vi "launch connection handler.vi"(7 "TCP Network Connection Refnum":refnum<k5>, 8 "error in":errorcluster, 9 "to application":refnum<queue>, 10 "to listener":refnum<queue>, 11 "VI ref":variant) -> (0 "error IO":errorcluster, 3 "to handler":refnum<queue>)   [LabVIEW 2015]
uses:
  message/message.ctl
  message/message type.lvlib
  TCP connection/TCP connection.lvclass
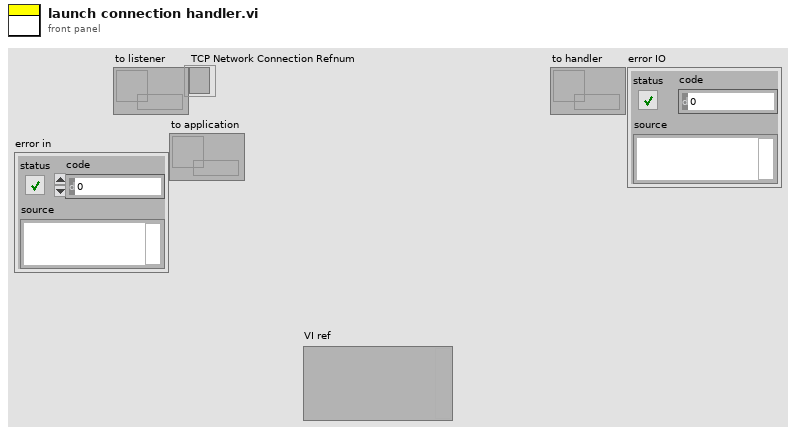
[diagram p1: front panel]
types:
  T1 = typedef "message type.lvlib/message.ctl" = cluster{"ID":string, "data":variant}
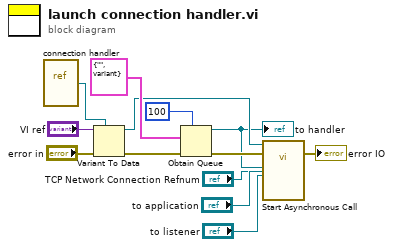
[diagram p0: block diagram]
diagram:
  n1 = vi-ref "connection handler.vi"() -> (w8:refnum<vi>)
  n2 = Variant To Data(error in="error in", type=w8, Variant="VI ref") -> (data=w6:refnum<vi>, error out=w9:errorcluster)
  n3 = Obtain Queue(max queue size (-1, unlimited)=100, element data type=T1 {"ID"="", "data"=variant} ("message"), error in (no error)=w9) -> (queue out=w5:refnum<queue>, error out=w11:errorcluster)  [unwired: 2 in, 1 out]
  "to handler" <- w5
  n4 = call-by-ref "Start Asynchronous Call"(reference=w6, error in=w11, "TCP Network Connection Refnum"="TCP Network Connection Refnum", "to application"="to application", "to listener"="to listener", "to handler"=w5) -> (error out=→"error IO":errorcluster)  [unwired: 8 in, 1 out]
